vi "Initialize.vi"(8 "error in (no error)":errorcluster, 11 "MFC in":refnum<class "Scale.lvclass">) -> (0 "error out":errorcluster, 3 "MFC out":refnum<class "Scale.lvclass">)   [LabVIEW 2013, in "Scale.lvlib" / "Scale.lvclass"]
uses:
  Scale.lvclass
  <vilib>/Instr/_visa.llb/VISA Configure Serial Port (Instr).vi
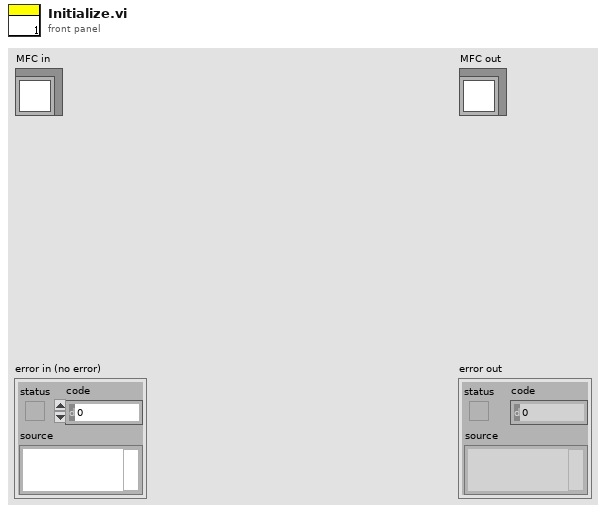
[diagram p1: front panel]
types:
  T1 = enum16{"open", "open or create", "create or replace", "create", "open (read-only)"}
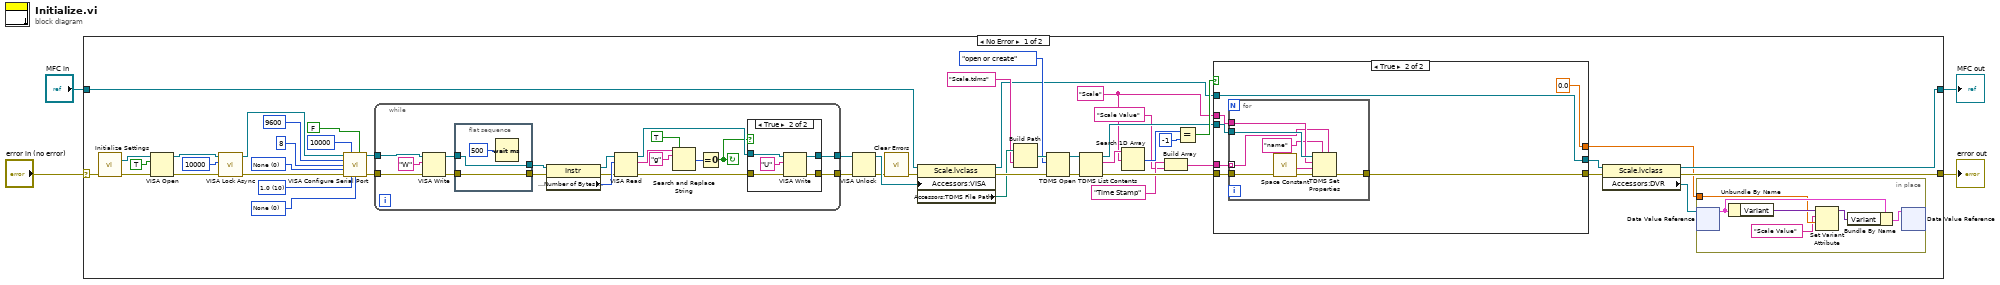
[diagram p0: block diagram]
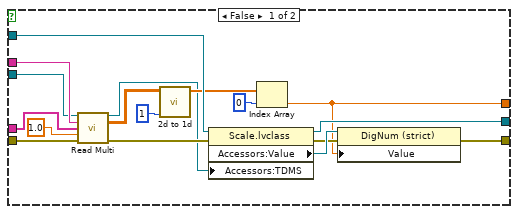
[diagram p3: hidden frame]
diagram:
  n1 = case shown="No Error" "error in (no error)" {
    selector: "error in (no error)" -> [w33 w120]
    tunnel: [w28 w120] -> w3
    tunnel: [w29 w119] -> w1
    tunnel: "MFC in" -> [w42 w119]
    frame No Error {
      w20 = u16 10 items=["1.0"=10, "1.5"=15, "2.0"=20] ("stop bits (10: 1 bit)")
      w18 = u16 0 items=["None", "Odd", "Even", "Mark", "Space"] ("parity")
      w19 = u16 0 items=["None"=0, "XON/XOFF"=1, "RTS/CTS"=2, "DTR/DSR"=4] ("flow control")
      w46 = "Scale"
      n2 = call "Initialize Settings.vi"("error in (no error)"=w33) -> ("VISA resource name 2"=w9:refnum<visa-resource-name>, "error out"=w10:errorcluster)  [unwired: 13 in]
      n3 = VISA Open(duplicate session (F)=TRUE, error in (no error)=w10, VISA resource name=w9) -> (VISA resource name=w23:refnum<visa-resource-name>, error out=w24:errorcluster)  [unwired: 2 in]
      n4 = call <vilib>:"VISA Lock Async.vi"("error in (no error)"=w24, "timeout (0)"=u32 10000, "VISA resource name"=w23) -> ("error out"=w13:errorcluster, "VISA resource name out"=w14:refnum<visa-resource-name>)  [unwired: 6 in, 1 out]
      n5 = call-poly "VISA Configure Serial Port"("VISA resource name"=w14, "timeout (10sec)"=u32 10000, "Enable Termination\nChar (T)"=FALSE ("Enable Termination Char (T)"), "baud rate (9600)"=u32 9600, "data bits (8)"=u16 8 ("data bits"), "parity (0:none)"=w18, "error in (no error)"=w13, "stop bits (10: 1 bit)"=w20, "flow control (0:none)"=w19) -> ("VISA resource name out"=w11:refnum<visa-resource-name>, "error out"=w12:errorcluster)  [unwired: 5 out]
      n6 = while {
        tunnel: w11 -> [w57]
        tunnel: w12 -> [w56]
        tunnel: [w55] -> w27
        tunnel: [w54] -> w26
        stop <- w53 continue-if-true
        n7 = VISA Write(VISA resource name=w57, write buffer="W", error in (no error)=w56) -> (VISA resource name out=w70:refnum<visa-resource-name>, error out=w69:errorcluster)  [unwired: 1 out]
        n8 = flat-sequence {
          tunnel: w70 -> [w81]
          tunnel: [w81] -> w58
          tunnel: [w80] -> w68
          tunnel: w69 -> [w80]
          frame #0 {
            n9 = Wait (ms)(milliseconds to wait=u32 500 ("ms before read")) -> ()  [unwired: 1 out]
          }
        }
        n10 = property class="Instr"(reference=w58, error in=w68) -> (reference out=w67:refnum<visa-resource-name>, error out=w65:errorcluster, "Serial Settings:Number of Bytes at Serial Port"=w66:u32)
        n11 = VISA Read(VISA resource name=w67, byte count=w66, error in (no error)=w65) -> (VISA resource name out=w59:refnum<visa-resource-name>, read buffer=w61:string, error out=w64:errorcluster)  [unwired: 1 out]
        n12 = Search and Replace String(replace all?=TRUE ("replace all? (F)"), input string=w61, search string="g" ("input string")) -> (number of replacements=w60:i32)  [unwired: 5 in, 3 out]
        n13 = Equal To 0?(x=w60) -> (x = 0?=w53:bool)
        n14 = case shown="True" w53 {
          tunnel: w64 -> [w73 w78]
          tunnel: w59 -> [w72 w77]
          tunnel: [w73 w74] -> w55
          tunnel: [w72 w75] -> w54
          frame False {
          }
          frame True {
            n15 = VISA Write(VISA resource name=w77, write buffer="U", error in (no error)=w78) -> (VISA resource name out=w75:refnum<visa-resource-name>, error out=w74:errorcluster)  [unwired: 1 out]
          }
        }
      }
      n16 = VISA Unlock(8:w27, 11:w26) -> (0:w7:errorcluster, 3:w8:refnum<visa-resource-name>)
      n17 = call <vilib>:"Clear Errors.vi"("error in (no error)"=w7) -> ("error out"=w6:errorcluster)  [unwired: 6 in]
      n18 = property class="Scale.lvclass"(reference=w42, error in=w6, "Accessors:VISA"=w8) -> (reference out=w34:refnum<class "Scale.lvclass">, error out=w40:errorcluster, "Accessors:TDMS File Path"=w37:path)
      n19 = Build Path(base path=w37, name or relative path="Scale.tdms") -> (appended path=w41:path)
      n20 = TDMS Open(8:w40, 10:T1."open or create" ("operation (0:open)"), 11:w41) -> (0:w39:errorcluster, 3:w35:refnum<k34>)  [unwired: 4 in]
      n21 = TDMS List Contents(4:w39, 7:w35) -> (0:w47:errorcluster, 2:w50:string[], 3:w48:refnum<k34>)  [unwired: 1 in, 1 out]
      n22 = Search 1D Array(1D array=w50, element=w46) -> (index of element=w51:i32)  [unwired: 1 in]
      n23 = Build Array("Time Stamp" ("Channel"), "Scale Value" ("string")) -> (w45:string[])
      n24 = Equal?(x=w51, y=-1) -> (x = y?=w49:bool)
      n25 = case shown="True" w49 {
        tunnel: w48 -> [w99 w111]
        tunnel: [w93 w107] -> w31
        tunnel: w47 -> [w102 w109]
        tunnel: w46 -> [w103 w110]
        tunnel: w34 -> [w104 w106]
        tunnel: w45 -> [w90 w108]
        tunnel: [w98 w106] -> w30
        tunnel: [w88 0.0 ("Numeric Control")] -> w5
        frame False {
          n26 = call "Read Multi.vi"("tdms file in"=w99, "group"=w103, "Channel"=w90, "Numeric"=1.0, "error in (no error)"=w102) -> ("tdms file out"=w91:refnum<k34>, "Array"=w96:dbl[][], "error out"=w101:errorcluster)  [unwired: 7 in, 1 out]
          n27 = call "2d to 1d.vi"("index"=1, "array"=w96) -> ("output array"=w95:dbl[])  [unwired: 9 in]
          n28 = property class="Scale.lvclass"(reference=w104, error in=w101, "Accessors:TDMS"=w91) -> (reference out=w98:refnum<class "Scale.lvclass">, error out=w89:errorcluster, "Accessors:Value"=w92:refnum<vi>)
          n29 = Index Array(array=w95, index=0) -> (element=w88:dbl)
          n30 = property class="DigNum (strict)"(reference=w92, error in=w89, "Value"=w88) -> (error out=w93:errorcluster)  [unwired: 1 out]
        }
        frame True {
          n31 = for {
            tunnel: w109 -> [w118]
            tunnel: [w117] -> w107
            tunnel: w111 -> [w116]
            tunnel: w110 -> [w115]
            tunnel: w108 -> [w114] mode=indexing
            n32 = call <vilib>:"Space Constant.vi"() -> ("String"=w112:string)
            n33 = TDMS Set Properties(5:w114, 7:"name" ("property names"), 8:w118, 9:w112, 10:w115, 11:w116) -> (0:w117:errorcluster)  [unwired: 3 out]
          }
        }
      }
      n34 = property class="Scale.lvclass"(reference=w30, error in=w31) -> (reference out=w29:refnum<class "Scale.lvclass">, error out=w28:errorcluster, "Accessors:DVR"=w32:refnum<data-value>)
      n35 = in-place {
        in-place-border: w5 -> [w83]
        n36 = in-place-dvr #1(w32) -> (w84:cluster{"Array":string[], "Variant":variant})  [unwired: 1 out]
        n37 = Unbundle By Name(w84) -> ("Variant"=w86:variant)
        n38 = Set Variant Attribute(Variant=w86, name="Scale Value" ("string"), value=w83) -> (Variant out=w85:variant)  [unwired: 1 in, 2 out]
        n39 = Bundle By Name(cluster=w84, "Variant"=w85) -> (w87:cluster{"Array":string[], "Variant":variant})
        n40 = in-place-dvr #1(w87) -> ()  [unwired: 2 out]
      }
    }
    frame Error {
    }
  }
  "error out" <- w3
  "MFC out" <- w1
